vi "Sending_FirmwareUpgrade_Cmd_SUB_VI.vi"(0 "Socket IP Address":string="192.168.1.100", 5 "Which one to upgrade?\nAC||PC||SC":string="1||1||1") -> (14 "AC":u8(slide) scale=0.0..100.0, 15 "PC":u8(slide) scale=0.0..100.0, 16 "SC":u8(slide) scale=0.0..100.0, 19 "error out":errorcluster)   [LabVIEW 2017]
panel:
  out "FW Upgrade Results":string="Horn Scan Success"
  out "connection ID out":refnum<k5>
  # "INPUT :"
  # "OUTPUT :"
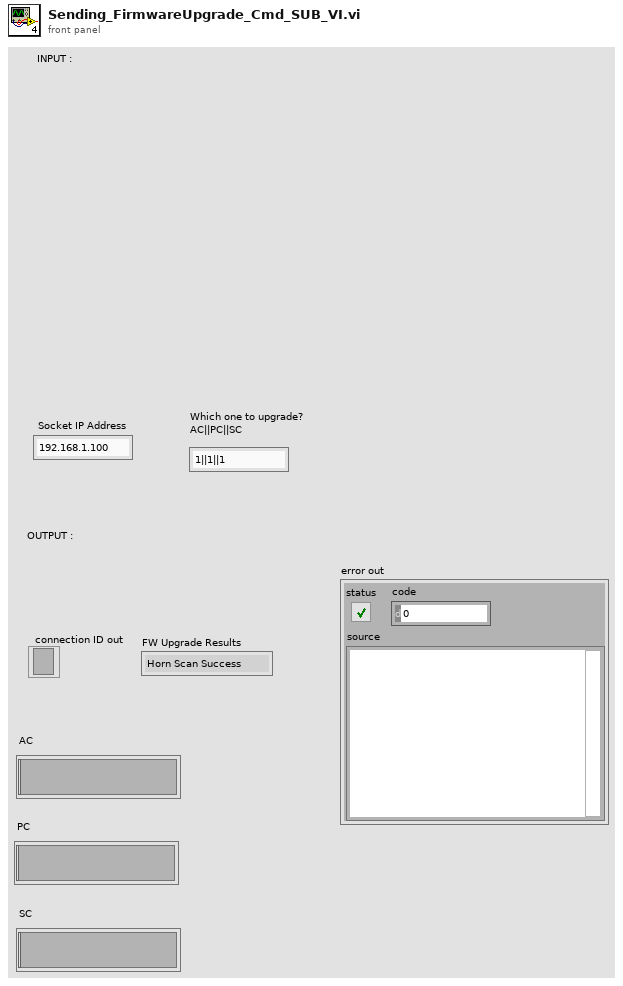
[diagram p1: front panel]
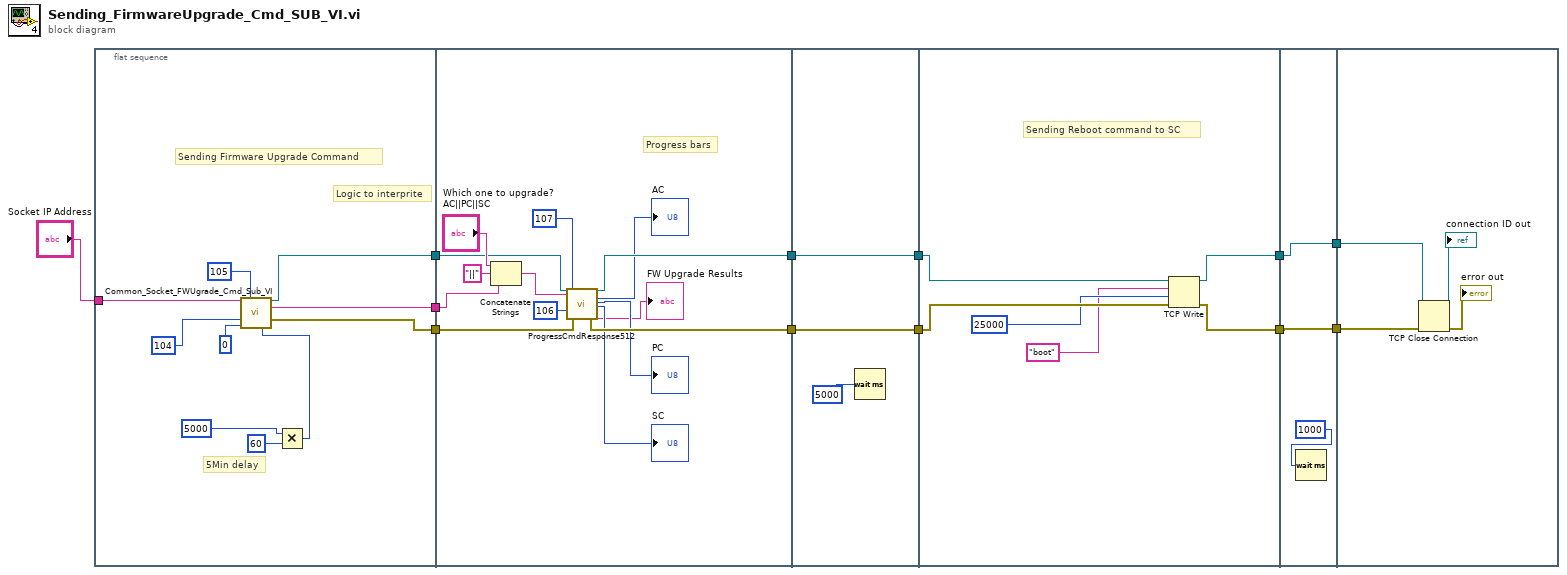
[diagram p0: block diagram]
diagram:
  n1 = flat-sequence {
    tunnel: [w22] -> w7
    tunnel: [w21] -> w5
    tunnel: "Socket IP Address" -> [w17]
    tunnel: [w13] -> w3
    tunnel: w7 -> [w32]
    tunnel: [w27] -> w6
    tunnel: w5 -> [w31]
    tunnel: [w30] -> w4
    tunnel: w3 -> [w35]
    tunnel: w6 -> [w39]
    tunnel: [w39] -> w12
    tunnel: w4 -> [w38]
    tunnel: [w38] -> w11
    tunnel: w12 -> [w44]
    tunnel: w11 -> [w45]
    tunnel: [w42] -> w10
    tunnel: [w43] -> w9
    tunnel: w10 -> [w47]
    tunnel: w9 -> [w46]
    tunnel: [w47] -> w2
    tunnel: [w46] -> w1
    tunnel: w2 -> [w50]
    tunnel: w1 -> [w49]
    frame #0 {
      # "Logic to interprite"
      # "5Min delay"
      # "Sending Firmware Upgrade Command"
      n2 = Multiply(x=i16 5000 ("Time Delay"), y=i16 60) -> (x*y=w15:i16)
      n3 = call "Common_Socket_FWUgrade_Cmd_Sub_VI.vi"("Socket IP Address"=w17, "Response ID 1"=u8 105, "FW Message ID"=104 ("Operation Message ID 1"), "FW Message Length"=0 ("Operation Message Length 1"), "Time Delay"=w15) -> ("connection ID"=w21:refnum<k5>, "Data Response"=w13:string, "error out"=w22:errorcluster)  [unwired: 7 in, 1 out]
    }
    frame #1 {
      # "Progress bars"
      n4 = Concatenate Strings("Which one to upgrade?\nAC||PC||SC", "||" ("string"), w35) -> (w33:string)
      n5 = call "ProgressCmdResponse512.vi"("connection ID control"=w31, "Command for FW upgrade"=w33, "FW Message ID"=106, "Response ID 1"=u8 107, "error in (no error)"=w32) -> ("connection ID"=w30:refnum<k5>, "AC-FW upgrade pregress bar"=→"AC":u8, "PC-FW upgrade pregress bar"=→"PC":u8, "SC-FW upgrade pregress bar"=→"SC":u8, "error out"=w27:errorcluster, "Pass"=→"FW Upgrade Results":string)  [unwired: 17 in]
    }
    frame #2 {
      n6 = Wait (ms)(milliseconds to wait=u32 5000) -> ()  [unwired: 1 out]
    }
    frame #3 {
      # "Sending Reboot command to SC"
      n7 = TCP Write(connection ID=w45, data in="boot", error in (no error)=w44, 9:25000 ("timeout ms (25000)")) -> (connection ID out=w42:refnum<k5>, error out=w43:errorcluster)  [unwired: 1 out]
    }
    frame #4 {
      n8 = Wait (ms)(milliseconds to wait=u32 1000) -> ()  [unwired: 1 out]
    }
    frame #5 {
      n9 = TCP Close Connection(connection ID=w50, error in (no error)=w49) -> (connection ID out=→"connection ID out":refnum<k5>, error out=→"error out":errorcluster)  [unwired: 1 in]
    }
  }
